vi "Open Hardware.vi"(8 "error in (no error)":errorcluster, 11 "Inst.AH2500 in":refnum<class "Inst.AH2500.lvclass">) -> (0 "error out":errorcluster, 3 "Inst.AH2500 out":refnum<class "Inst.AH2500.lvclass">)   [LabVIEW 2019, in "Inst.AH2500.lvclass"]
uses:
  Inst.AH2500.lvclass
  C:/Program Files (x86)/National Instruments/LabVIEW 2019/user.lib/LevyLab/Instrument Framework/SMOs/Instrument/Instrument.lvclass
  <userlib>/LevyLab/Instrument Framework/SMOs/Instrument/Instrument.lvclass/Instrument.ctl
  Inst.AH2500.lvclass/Inst.AH2500.ctl
  <userlib>/LevyLab/Instrument Framework/Instrument Types/VSource/Instrument.VSource.lvclass
  <userlib>/LevyLab/Instrument Framework/SMOs/Instrument/Instrument.lvclass
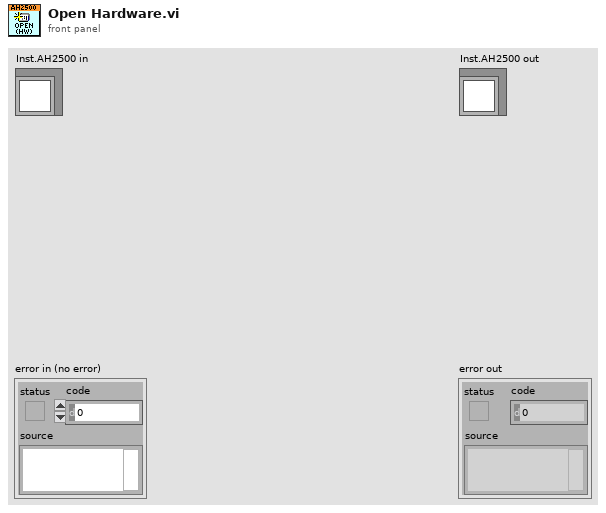
[diagram p1: front panel]
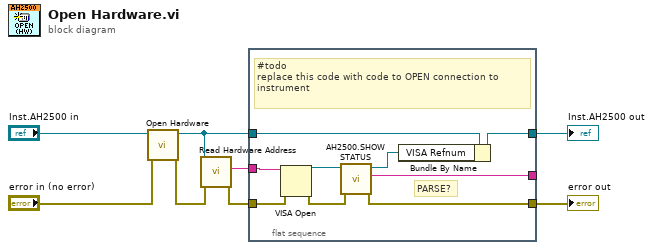
[diagram p0: block diagram]
diagram:
  n1 = call-parent "Open Hardware.vi"("error in (no error)"="error in (no error)", "Instrument in"="Inst.AH2500 in") -> ("error out"=w6:errorcluster, "Instrument out"=w5:refnum<class "Inst.AH2500.lvclass">)  [unwired: 8 in]
  n2 = call <userlib>:"Read Hardware Address.vi"("error in (no error)"=w6, "Instrument in"=w5) -> ("error out"=w3:errorcluster, "Address"=w1:string)  [unwired: 7 in, 1 out]
  n3 = flat-sequence {
    tunnel: w5 -> [w17]
    tunnel: [w16] -> w4
    tunnel: w3 -> [w15]
    tunnel: [w10] -> w2
    tunnel: w1 -> [w14]
    tunnel: [w9] -> _
    frame #0 {
      # "PARSE?"
      # "#todo\nreplace this code with code to OPEN connection to instrument"
      n4 = VISA Open(error in (no error)=w15, VISA resource name=w14) -> (VISA resource name=w13:refnum<visa-resource-name>, error out=w11:errorcluster)  [unwired: 3 in]
      n5 = call "AH2500.SHOW STATUS.vi"("error in (no error)"=w11, "VISA resource name"=w13) -> ("error out"=w10:errorcluster, "read buffer"=w9:string, "VISA resource name out"=w12:refnum<visa-resource-name>)  [unwired: 7 in]
      n6 = Bundle By Name(cluster=w17, "VISA Refnum"=w12) -> (w16:refnum<class "Inst.AH2500.lvclass">)
    }
  }
  "error out" <- w2
  "Inst.AH2500 out" <- w4
